vi "Alternating LEDs.vi"() -> ()   [LabVIEW 2015]
panel:
  out "LED 2":bool
  out "LED 1":bool
  in  "stop":bool
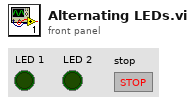
[diagram p1: front panel]
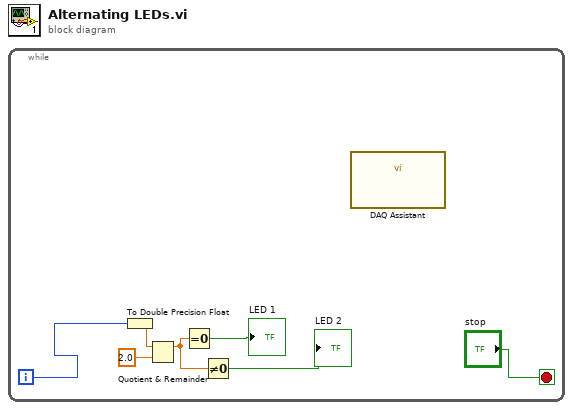
[diagram p0: block diagram]
diagram:
  n1 = while {
    i -> [w5]
    stop <- "stop" stop-if-true
    n2 = To Double Precision Float(number=w5) -> (double precision float=w6:dbl)
    n3 = Quotient & Remainder(x=w6, y=2.0) -> (x-y*floor(x/y)=w3:dbl)  [unwired: 1 out]
    n4 = Equal To 0?(x=w3) -> (x = 0?=→"LED 1":bool)
    n5 = Not Equal To 0?(x=w3) -> (x != 0?=→"LED 2":bool)
    n6 = call "DAQ Assistant"() -> ()  [unwired: 12 in]
  }
